vi "zeta_f(tau)_Analytical.vi"(6 "t0":ext, 7 "Harmonic f":ext, 11 "tau":ext) -> (3 "z":cxt)   [LabVIEW 2019]
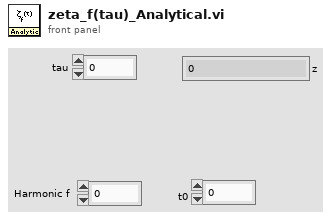
[diagram p1: front panel]
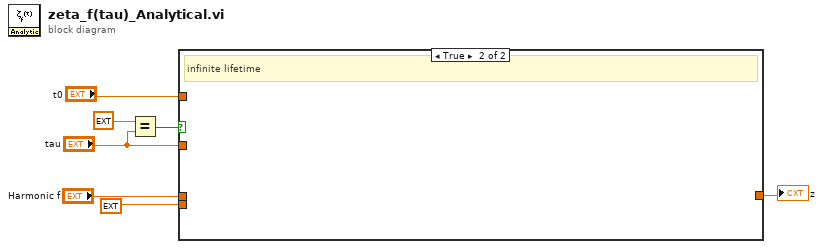
[diagram p0: block diagram]
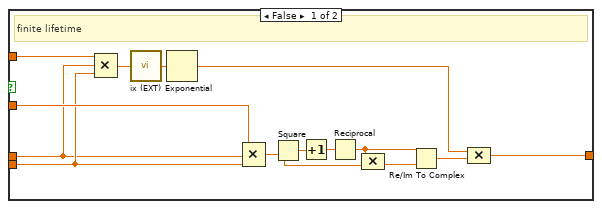
[diagram p2: hidden frame]
diagram:
  n1 = Equal?(x=ext inf ("y"), y="tau") -> (x = y?=w3:bool)
  n2 = case shown="True" w3 {
    tunnel: "Harmonic f" -> [w12 _]
    tunnel: ext 6.283185307179586477 -> [w13 _]
    tunnel: "t0" -> [w14 _]
    tunnel: "tau" -> [w18 _]
    tunnel: [w10 _] -> w1
    frame False {
      # "x exp(i 2 pi f t_0)"
      # "finite lifetime"
      n3 = Compound Arithmetic op=MULTIPLY(w14, w12, w13) -> (w9:ext)
      n4 = call "ix (EXT).vi"("x (1)"=w9) -> ("ix"=w8:cxt)
      n5 = Exponential(1:w8) -> (0:w11:cxt)
      n6 = Compound Arithmetic op=MULTIPLY(w18, w12, w13) -> (w19:ext)
      n7 = Square(x=w19) -> (x^2=w20:ext)
      n8 = Increment(x=w20) -> (x+1=w21:ext)
      n9 = Reciprocal(x=w21) -> (1/x=w17:ext)
      n10 = Compound Arithmetic op=MULTIPLY(w17, w19) -> (w16:ext)
      n11 = Re/Im To Complex(1:w16, 2:w17) -> (0:w15:cxt)
      n12 = Compound Arithmetic op=MULTIPLY(w11, w15) -> (w10:cxt)
    }
    frame True {
      # "infinite lifetime"
    }
  }
  "z" <- w1
